vi "Prosilica Q2D Calibration and acquisition.vi"() -> ()   [LabVIEW 2012]
uses:
  <vilib>/userdefined/High Color/IMAQdx.ctl
  <vilib>/vision/driver/IMAQdx.llb/IMAQdx Acquisition Mode.ctl
  <vilib>/vision/driver/IMAQdx.llb/IMAQdx Buffer Number Mode.ctl
  <resource>/objmgr/imaqdx.rc
  <vilib>/vision/driver/NI_Vision_Acquisition_Software.lvlib
  Program Files/Mad City Labs/NanoDrive/Labview Examples/Madlib.dll
panel:
  in  "Stop Acquisition":bool
  out "Image":T1(plugin-control)
  in  "Desired Z Position":dbl=100.0 min=0.0 max=200.0 step=0.01 format="%.4f"
  in  "Desired Y Position":dbl=100.0 min=0.0 max=200.0 step=0.1 format="%.4f"
  out "Current Z Position (um)":dbl format="%.2f"
  out "Current Y Position (um)":dbl format="%.2f"
  in  "Desire X Position":dbl=100.0 min=0.0 max=200.0 step=0.1 format="%.4f"
  out "Current X Position (um)":dbl format="%.2f"
  out "Acquisition  progress":i32(slide) scale=0.0..2999.0
  in  "BitsPerPixel":u32(ring) items=["Use Hardware Value"=0, "10-bit"=10, "12-bit"=12, "14-bit"=14, "16-bit"=16]
  in  "Height":u32=1080
  in  "Width":u32=1920
  in  "Path 2":path
  in  "Exposure":dbl(slide)=1407.017543859649 min=100.0 max=15000.0 step=100.0 scale=100.0..15000.0
  in  "Stop VI":bool
  in  "Start Acquisition":bool
  in  "Number of Frames":u32=3000
  in  "Frame Rate":dbl=55.0
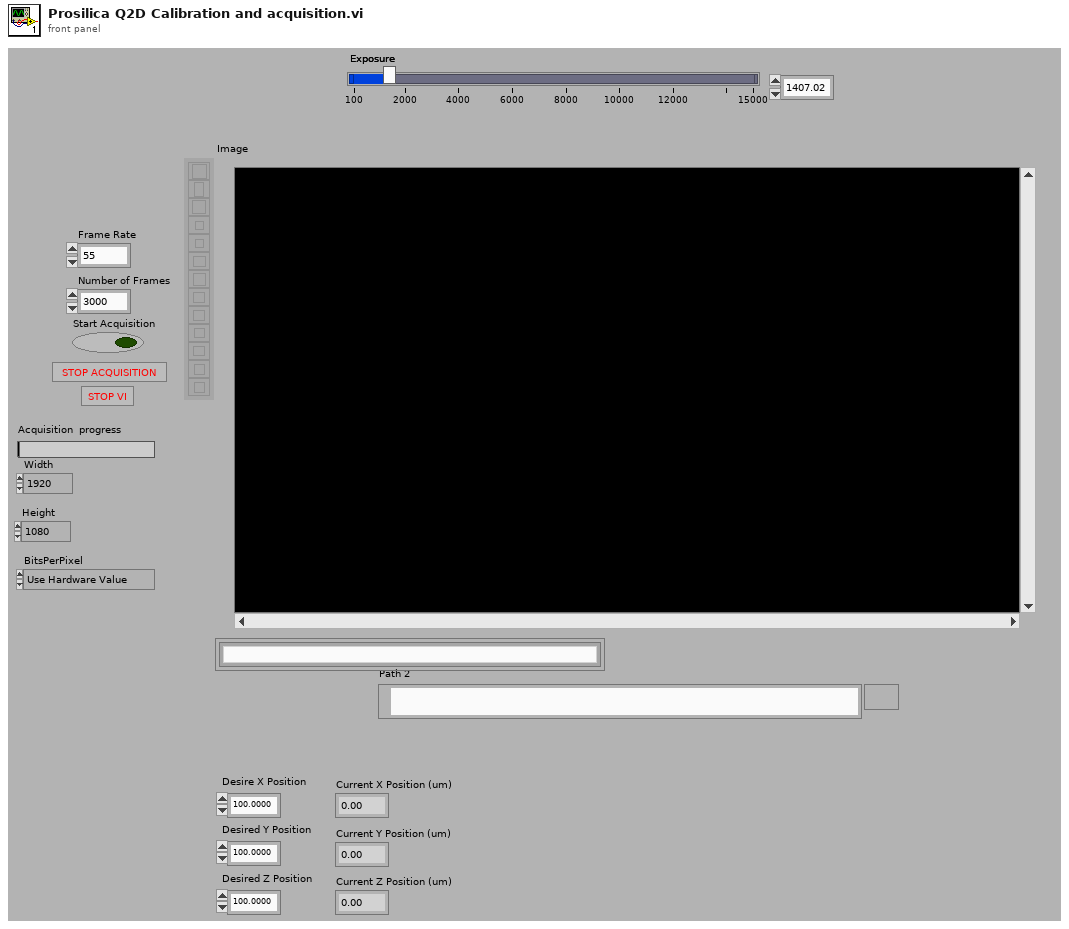
[diagram p1: front panel]
types:
  T1 = typedef "IMAQ Image.ctl" = refnum<image>
  T2 = typedef "IMAQdx.ctl" = refnum<k21>
  T3 = typedef "NI_Vision_Acquisition_Software.lvlib/IMAQdx Buffer Number Mode.ctl" = enum32{"Next", "Last", "Buffer Number"}
  T4 = typedef "NI_Vision_Acquisition_Software.lvlib/IMAQdx Acquisition Mode.ctl" = enum32{"One Shot", "Continuous"}
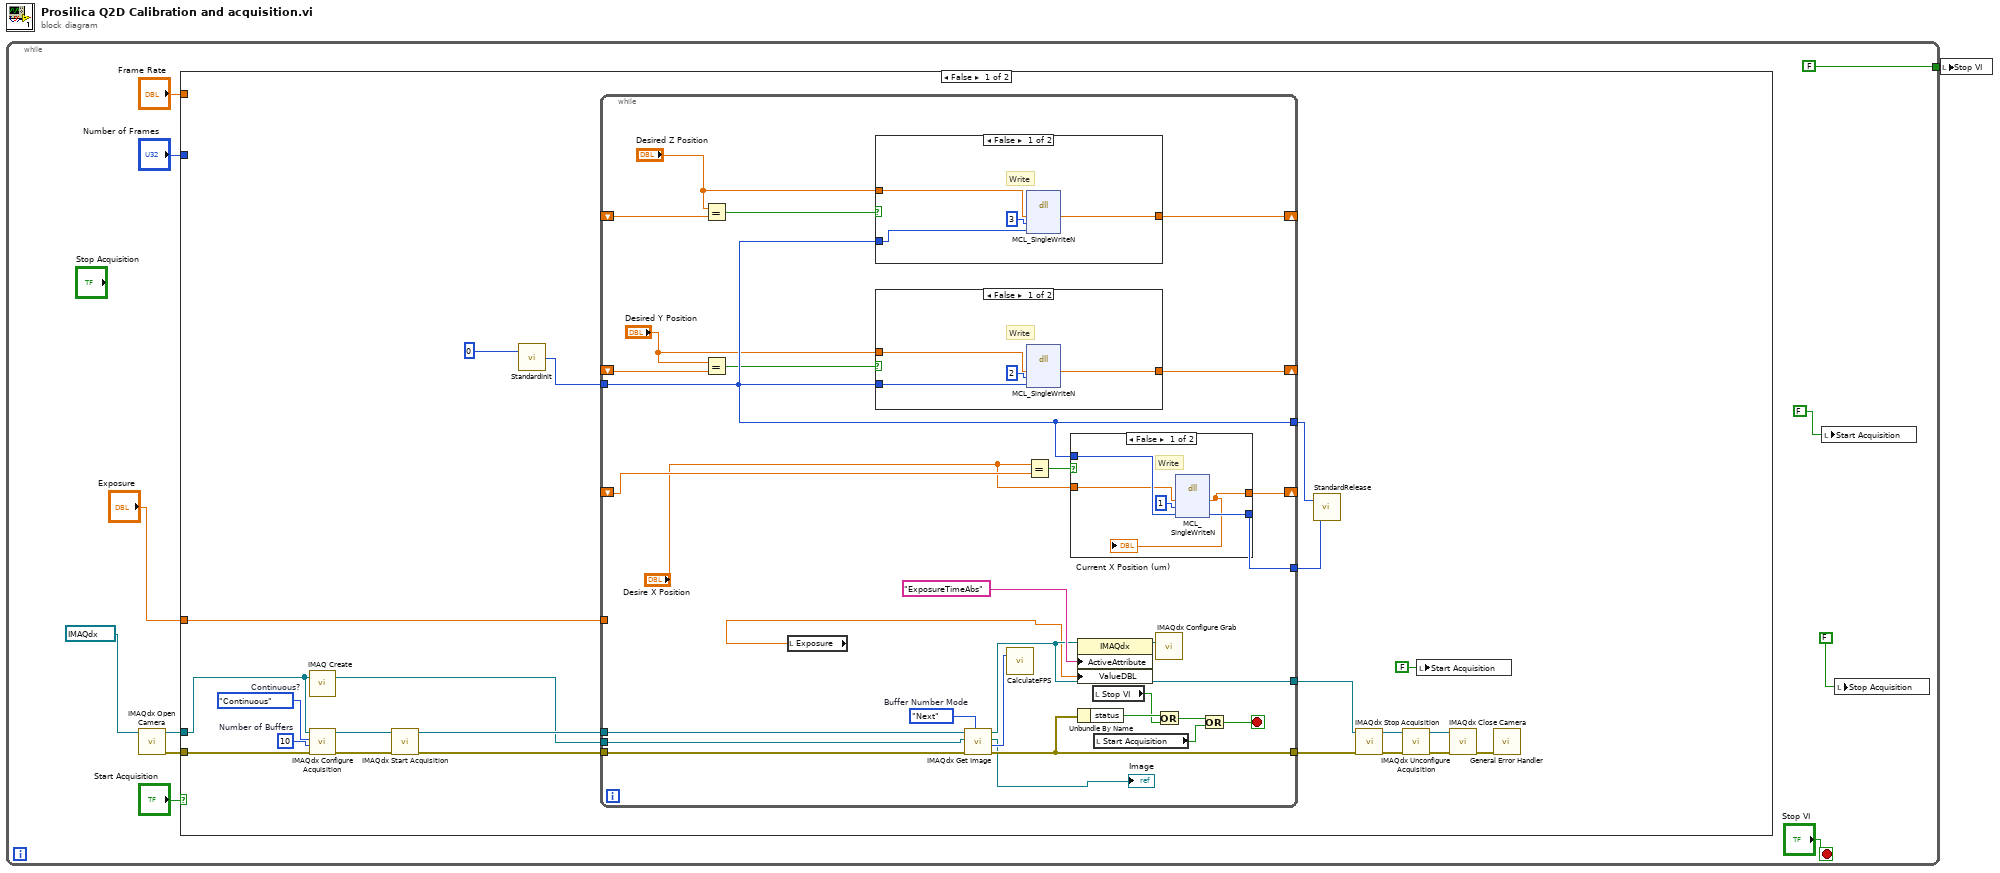
[diagram p0: block diagram]
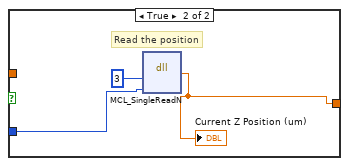
[diagram p2: hidden frame]
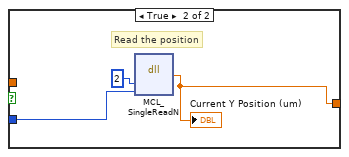
[diagram p3: hidden frame]
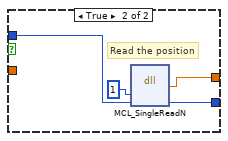
[diagram p4: hidden frame]
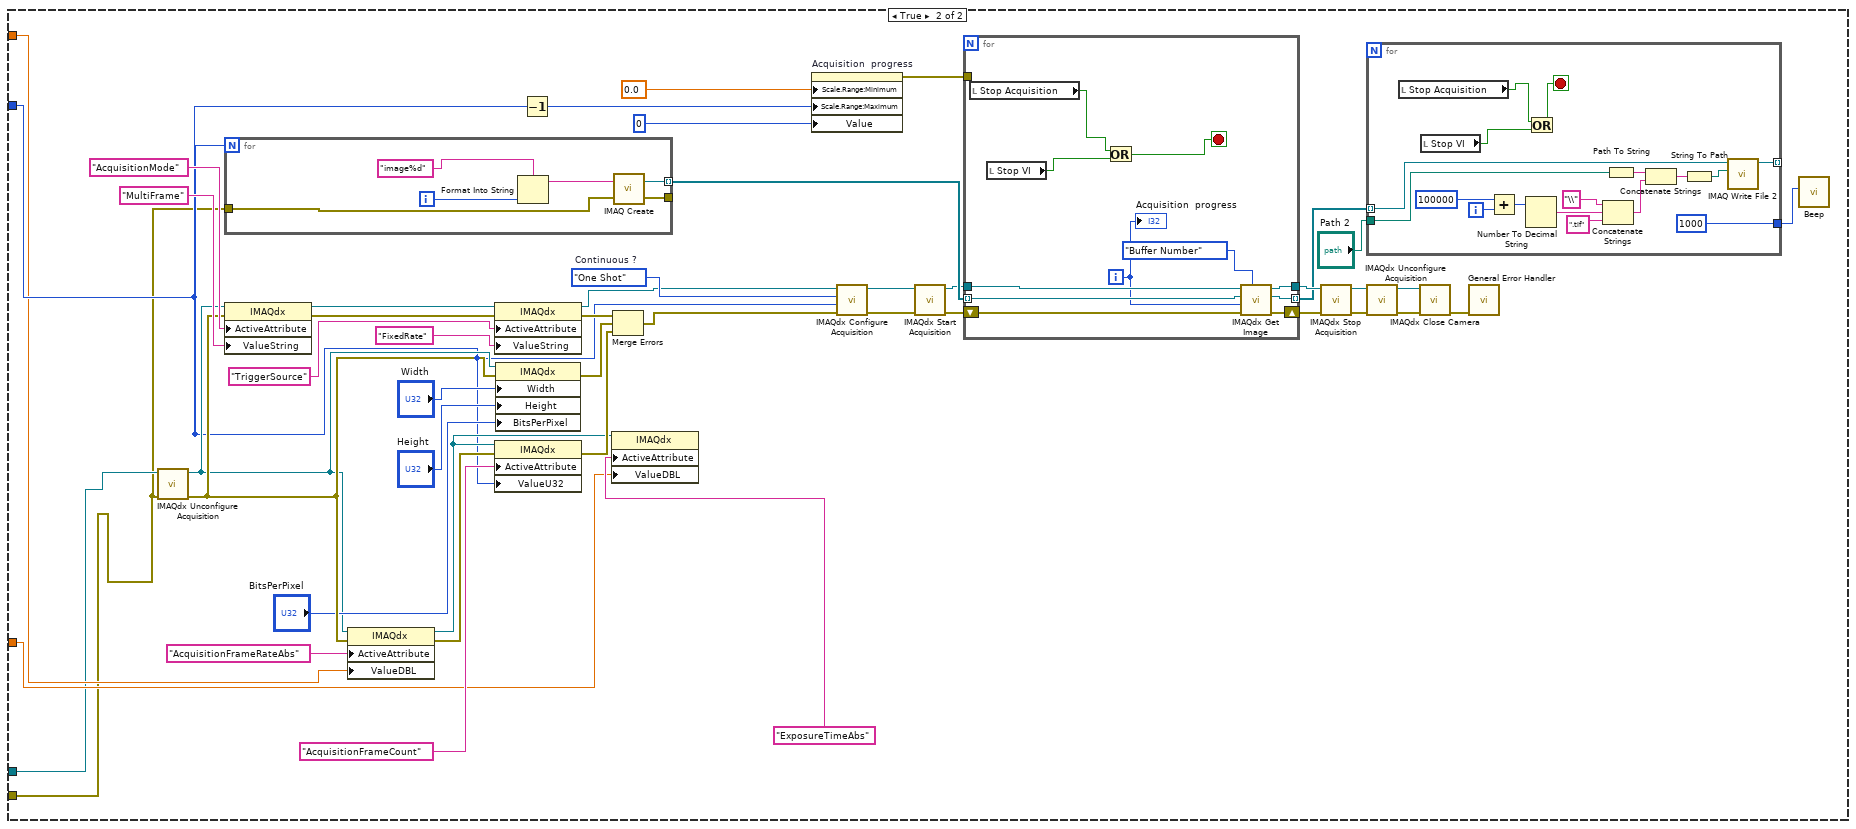
[diagram p5: hidden frame]
diagram:
  n1 = while {
    tunnel: [FALSE] -> w1
    stop <- "Stop VI" stop-if-true
    n2 = call <vilib>:"IMAQdx Open Camera.vi"("Session In"=T2 "cam0") -> ("error out"=w7:errorcluster, "Session Out"=w8:T2)  [unwired: 2 in, 7 out]
    n3 = case shown="False" "Start Acquisition" {
      tunnel: "Frame Rate" -> [_ w92]
      tunnel: "Number of Frames" -> [_ w93]
      tunnel: w8 -> [w25 w90]
      tunnel: w7 -> [w24 w89]
      tunnel: "Exposure" -> [w16 w91]
      frame False {
        w31 = IMAQdx_Acquisition_Mode."Continuous"  # Continuous?
        w30 = u32 10  # Number of Buffers
        n4 = call "IMAQ Create"("Image Name"=w25) -> ("New Image"=w19:T1)  [unwired: 3 in, 2 out]
        n5 = call <vilib>:"IMAQdx Configure Acquisition.vi"("error in"=w24, "Number of Buffers"=w30, "Continuous?"=w31, "Session In"=w25) -> ("error out"=w32:errorcluster, "Session Out"=w33:T2)  [unwired: 6 out]
        n6 = call <vilib>:"IMAQdx Start Acquisition.vi"("error in"=w32, "Session In"=w33) -> ("error out"=w23:errorcluster, "Session Out"=w22:T2)  [unwired: 8 out]
        n7 = call "StandardInit.vi"("Incoming Handle"=0) -> ("Outgoing Handle"=w14:i32)
        n8 = while {
          tunnel: w23 -> [w62]
          tunnel: w22 -> [w61]
          tunnel: [w42] -> w21
          tunnel: [w60] -> w20
          tunnel: w19 -> [w59]
          shift-right: [w40] -> _
          shift-left: _ -> [w41]
          tunnel: w14 -> [w49]
          tunnel: [w52] -> w18
          tunnel: [w49] -> w17
          shift-right: [w51] -> _
          shift-left: _ -> [w48]
          shift-right: [w50] -> _
          shift-left: _ -> [w46]
          tunnel: w16 -> [_]
          stop <- w54 stop-if-true
          w63 = IMAQdx_Buffer_Number_Mode."Next"  # Buffer Number Mode
          n9 = Equal?(x="Desired Z Position", y=w46) -> (x = y?=w45:bool)
          n10 = Equal?(x="Desired Y Position", y=w48) -> (x = y?=w47:bool)
          n11 = local read "Exposure"() -> (w35:dbl)
          n12 = case shown="False" w45 {
            tunnel: [w67 w69] -> w50
            tunnel: w49 -> [w66 w70]
            tunnel: "Desired Z Position" -> [w65 _]
            frame False {
              # "Write"
              n13 = dll-call lib="C:/Program Files/Mad City Labs/NanoDrive/Labview Examples/Madlib.dll" fn="MCL_SingleWriteN"("position"=w65, "axis"=u32 3, "handle"=w66) -> ("position"=w67:dbl)  [unwired: 5 in, 3 out]
            }
            frame True {
              # "Read the position"
              n14 = dll-call lib="C:/Program Files/Mad City Labs/NanoDrive/Labview Examples/Madlib.dll" fn="MCL_SingleReadN"("axis"=u32 3, "handle"=w70) -> (w69:dbl)  [unwired: 5 in, 2 out]
              "Current Z Position (um)" <- w69
            }
          }
          n15 = case shown="False" w47 {
            tunnel: [w74 w76] -> w51
            tunnel: w49 -> [w73 w77]
            tunnel: "Desired Y Position" -> [w72 _]
            frame False {
              # "Write"
              n16 = dll-call lib="C:/Program Files/Mad City Labs/NanoDrive/Labview Examples/Madlib.dll" fn="MCL_SingleWriteN"("position"=w72, "axis"=u32 2, "handle"=w73) -> ("position"=w74:dbl)  [unwired: 5 in, 3 out]
            }
            frame True {
              # "Read the position"
              n17 = dll-call lib="C:/Program Files/Mad City Labs/NanoDrive/Labview Examples/Madlib.dll" fn="MCL_SingleReadN"("axis"=u32 2, "handle"=w77) -> ("return type"=w76:dbl)  [unwired: 5 in, 2 out]
              "Current Y Position (um)" <- w76
            }
          }
          n18 = call <vilib>:"IMAQdx Get Image.vi"("Buffer Number Mode (Next)"=w63, "error in"=w62, "Image In"=w59, "Session In"=w61) -> ("error out"=w60:errorcluster, "Buffer Number Out"=w58:u32, "Image Out"=→"Image":T1, "Session Out"=w42:T2)  [unwired: 1 in, 3 out]
          n19 = call "CalculateFPS.vi"("buffer number"=w58) -> ()  [unwired: 3 out]
          n20 = Equal?(x="Desire X Position", y=w41) -> (x = y?=w53:bool)
          n21 = case shown="False" w53 {
            tunnel: w49 -> [w82 w86]
            tunnel: [w81 w85] -> w52
            tunnel: [w80 w84] -> w40
            tunnel: "Desire X Position" -> [w79 _]
            frame False {
              # "Write"
              n22 = dll-call lib="C:/Program Files/Mad City Labs/NanoDrive/Labview Examples/Madlib.dll" fn="MCL_SingleWriteN"("position"=w79, "axis"=u32 1, "handle"=w82) -> ("position"=w80:dbl, "handle"=w81:i32)  [unwired: 4 in, 3 out]
              "Current X Position (um)" <- w80
            }
            frame True {
              # "Read the position"
              n23 = dll-call lib="C:/Program Files/Mad City Labs/NanoDrive/Labview Examples/Madlib.dll" fn="MCL_SingleReadN"("axis"=u32 1, "handle"=w86) -> ("return type"=w84:dbl, "handle"=w85:i32)  [unwired: 4 in, 2 out]
            }
          }
          n24 = property class="IMAQdx"(reference=w42, "ActiveAttribute"="ExposureTimeAbs", "ValueDBL"=w35) -> (reference out=w43:T2)  [unwired: 1 in, 1 out]
          n25 = Unbundle By Name(w60) -> ("status"=w64:bool)
          n26 = local read "Stop VI"() -> (w57:bool)
          n27 = local read "Start Acquisition"() -> (w56:bool)
          n28 = call <vilib>:"IMAQdx Configure Grab.vi"("Session In"=w43) -> ()  [unwired: 9 in, 2 out]
          n29 = Or(x=w64, y=w57) -> (x .or. y?=w55:bool)
          n30 = Or(x=w55, y=w56) -> (x .or. y?=w54:bool)
        }
        n31 = call "StandardRelease.vi"("Outgoing Handle"=w18, "Incoming Handle"=w17) -> ()  [unwired: 1 out]
        n32 = call <vilib>:"IMAQdx Stop Acquisition.vi"("error in"=w20, "Session In"=w21) -> ("error out"=w26:errorcluster, "Session Out"=w27:T2)  [unwired: 8 out]
        n33 = call <vilib>:"IMAQdx Unconfigure Acquisition.vi"("error in"=w26, "Session In"=w27) -> ("error out"=w29:errorcluster, "Session Out"=w28:T2)  [unwired: 8 out]
        n34 = local write "Start Acquisition"(FALSE ("Start Acquisition")) -> ()
        n35 = call <vilib>:"IMAQdx Close Camera.vi"("error in"=w29, "Session In"=w28) -> ("error out"=w34:errorcluster)  [unwired: 9 out]
        n36 = call <vilib>:"General Error Handler.vi"("error in (no error)"=w34) -> ()  [unwired: 1 in, 14 out]
      }
      frame True {
        w115 = IMAQdx_Acquisition_Mode."One Shot"  # Continuous ?
        n37 = call <vilib>:"IMAQdx Unconfigure Acquisition.vi"("error in"=w89, "Session In"=w90) -> ("error out"=w120:errorcluster, "Session Out"=w117:T2)  [unwired: 8 out]
        n38 = for {
          N: w93 -> [_]
          tunnel: w89 -> [w167]
          tunnel: [w166] -> w103 mode=indexing
          tunnel: [w165] -> _
          i -> [w164]
          n39 = Format Into String(format string="image%d" ("Image Name"), w164) -> (resulting string=w163:string)  [unwired: 2 in, 1 out]
          n40 = call "IMAQ Create"("Image Name"=w163, "error in (no error)"=w167) -> ("New Image"=w166:T1, "error out"=w165:errorcluster)  [unwired: 2 in, 1 out]
        }
        n41 = property class="IMAQdx"(reference=w117, error in=w120, "ActiveAttribute"="AcquisitionMode", "ValueString"="MultiFrame") -> (reference out=w121:T2, error out=w128:errorcluster)
        n42 = property class="IMAQdx"(reference=w117, error in=w120, "ActiveAttribute"="AcquisitionFrameRateAbs", "ValueDBL"=w92) -> (reference out=w94:T2, error out=w131:errorcluster)
        n43 = property class="IMAQdx"(reference=w121, error in=w128, "ActiveAttribute"="TriggerSource", "ValueString"="FixedRate") -> (reference out=w102:T2, error out=w124:errorcluster)
        n44 = property class="IMAQdx"(reference=w94, error in=w131, "ActiveAttribute"="AcquisitionFrameCount", "ValueU32"=w93) -> (error out=w125:errorcluster)  [unwired: 1 out]
        n45 = property class="IMAQdx"(reference=w117, error in=w120, "Width"="Width", "Height"="Height", "BitsPerPixel"="BitsPerPixel") -> (error out=w119:errorcluster)  [unwired: 1 out]
        n46 = Decrement(x=w93) -> (x-1=w112:u32)
        n47 = property class="IMAQdx"(reference=w94, "ActiveAttribute"="ExposureTimeAbs", "ValueDBL"=w91) -> ()  [unwired: 1 in, 2 out]
        n48 = Merge Errors(w124, w119, w125) -> (w99:errorcluster)
        n49 = property on="Acquisition  progress" class="Slide (strict)"("Scale.Range:Minimum"=0.0 ("Write Attribute"), "Scale.Range:Maximum"=w112, "Value"=u32 0 ("Acquisition  progress")) -> (error out=w104:errorcluster)  [unwired: 2 in, 1 out]
        n50 = call <vilib>:"IMAQdx Configure Acquisition.vi"("error in"=w99, "Number of Buffers"=w93, "Continuous?"=w115, "Session In"=w102) -> ("error out"=w98:errorcluster, "Session Out"=w101:T2)  [unwired: 6 out]
        n51 = call <vilib>:"IMAQdx Start Acquisition.vi"("error in"=w98, "Session In"=w101) -> ("error out"=w114:errorcluster, "Session Out"=w100:T2)  [unwired: 8 out]
        n52 = for {
          tunnel: w103 -> [w161] mode=indexing
          shift-right: [w159] -> w111
          shift-left: w114 -> [w160]
          tunnel: [w158] -> w110
          tunnel: w100 -> [w157]
          tunnel: [w154] -> w96 mode=indexing
          tunnel: w104 -> [_]
          i -> [w155]
          stop <- w151 stop-if-true
          n53 = local read "Stop Acquisition"() -> (w153:bool)
          n54 = local read "Stop VI"() -> (w152:bool)
          n55 = Or(x=w153, y=w152) -> (x .or. y?=w151:bool)
          n56 = call <vilib>:"IMAQdx Get Image.vi"("Buffer Number Mode (Next)"=IMAQdx_Buffer_Number_Mode."Buffer Number", "error in"=w160, "Buffer Number In"=w155, "Image In"=w161, "Session In"=w157) -> ("error out"=w159:errorcluster, "Image Out"=w154:T1, "Session Out"=w158:T2)  [unwired: 4 out]
          "Acquisition  progress" <- w155
        }
        n57 = call <vilib>:"IMAQdx Stop Acquisition.vi"("error in"=w111, "Session In"=w110) -> ("error out"=w109:errorcluster, "Session Out"=w108:T2)  [unwired: 8 out]
        n58 = for {
          tunnel: "Path 2" -> [w140]
          tunnel: w96 -> [w139] mode=indexing
          tunnel: [w138] -> _ mode=indexing
          tunnel: [1000] -> w88
          i -> [w145]
          stop <- w135 stop-if-true
          n59 = local read "Stop Acquisition"() -> (w136:bool)
          n60 = local read "Stop VI"() -> (w137:bool)
          n61 = Add(x=100000, y=w145) -> (x+y=w147:i32)
          n62 = Number To Decimal String(number=w147) -> (decimal integer string=w150:string)  [unwired: 1 out]
          n63 = Or(x=w136, y=w137) -> (x .or. y?=w135:bool)
          n64 = Concatenate Strings("\\" ("string"), w150, ".tif") -> (w142:string)
          n65 = Path To String(path=w140) -> (string=w144:string)
          n66 = Concatenate Strings(w144, w142) -> (w143:string)
          n67 = String To Path(string=w143) -> (path=w141:path)
          n68 = call-poly "IMAQ Write File 2"("File Path"=w141, "Image"=w139) -> ("Image Out (duplicate)"=w138:T1)  [unwired: 3 in, 6 out]
        }
        n69 = call <vilib>:"IMAQdx Unconfigure Acquisition.vi"("error in"=w109, "Session In"=w108) -> ("error out"=w107:errorcluster, "Session Out"=w106:T2)  [unwired: 8 out]
        n70 = call <vilib>:"IMAQdx Close Camera.vi"("error in"=w107, "Session In"=w106) -> ("error out"=w116:errorcluster)  [unwired: 9 out]
        n71 = call <vilib>:"General Error Handler.vi"("error in (no error)"=w116) -> ()  [unwired: 1 in, 14 out]
        n72 = call <vilib>:"Beep.vi"("duration (msec)"=w88) -> ()  [unwired: 11 in]
      }
    }
    n73 = local write "Start Acquisition"(FALSE ("Start Acquisition")) -> ()
    n74 = local write "Stop Acquisition"(FALSE ("Stop Acquisition")) -> ()
  }
  n75 = local write "Stop VI"(w1) -> ()
